vi "raise to negative two thirds.vi"(4 "Numeric in":dbl) -> (1 "Numeric out":dbl)   [LabVIEW 2019]
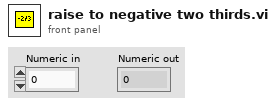
[diagram p1: front panel]
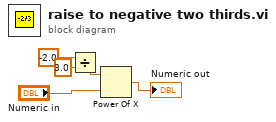
[diagram p0: block diagram]
diagram:
  n1 = Divide(x=-2.0, y=3.0) -> (x/y=w1:dbl)
  n2 = Power Of X(1:"Numeric in", 2:w1) -> (0:→"Numeric out":dbl)
